vi "ExecutionFrequencyHistory.vi"(11 "History Length":i32) -> (1 "TimestampHistory (s)":dbl[](array[numeric]), 2 "FrequencyHistory (s)":dbl[](array[numeric]), 3 "PeriodHistory (s)":dbl[](array[numeric]))   [LabVIEW 2014]
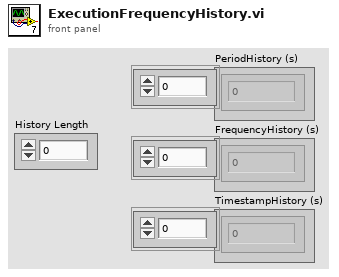
[diagram p1: front panel]
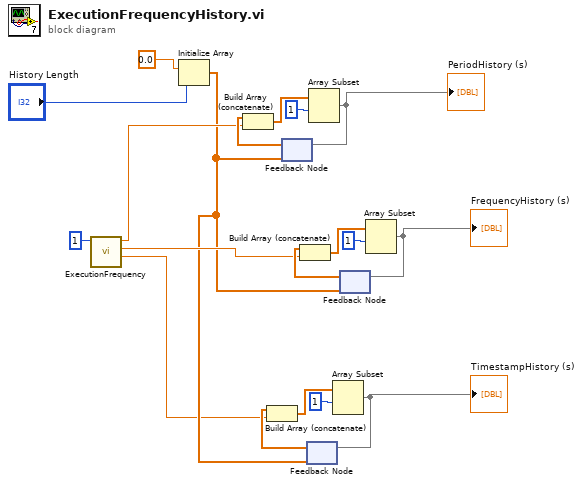
[diagram p0: block diagram]
diagram:
  n1 = call "ExecutionFrequency.vi"("Moving Average Length"=1) -> ("Timestamp (s)"=w2:dbl, "Frequency (Hz)"=w8:dbl, "Period (s)"=w13:dbl)  [unwired: 8 in]
  n2 = Initialize Array(0.0 ("élément"), "History Length") -> (w3:dbl[])
  n3 = feedback #1(w3) -> (w19:dbl[])
  n4 = Build Array (concatenate)(w19, w13) -> (w18:dbl[])
  n5 = feedback #2(w3) -> (w6:dbl[])
  n6 = Build Array (concatenate)(w6, w2) -> (w5:dbl[])
  n7 = Array Subset(array=w18, index=1) -> (w14:dbl[])  [unwired: 1 in]
  "PeriodHistory (s)" <- w14
  n8 = feedback-in #1(w14) -> ()
  n9 = Array Subset(array=w5, index=1) -> (w7:dbl[])  [unwired: 1 in]
  "TimestampHistory (s)" <- w7
  n10 = feedback-in #2(w7) -> ()
  n11 = feedback #3(w3) -> (w10:dbl[])
  n12 = Build Array (concatenate)(w10, w8) -> (w11:dbl[])
  n13 = Array Subset(array=w11, index=1) -> (w9:dbl[])  [unwired: 1 in]
  "FrequencyHistory (s)" <- w9
  n14 = feedback-in #3(w9) -> ()
